vi "ILCTemperatureOnly.vi"() -> ()   [LabVIEW 2016]
uses:
  Common_RT_HealthAndStatus/RTHealthAndStatus/RTHealthAndStatus.lvclass
  MyHealthAndStatusReadFIFO/MyHealthAndStatusReadFIFO.lvclass
  D:/Code/Common_RT_FPGA/IReadU32FIFO/IReadU32FIFO.lvclass
  MyHealthAndStatusWriteFIFO/MyHealthAndStatusWriteFIFO.lvclass
  D:/Code/Common_RT_FPGA/IWriteU64FIFO/IWriteU64FIFO.lvclass
  ModbusFactory/ModbusFactory.lvclass
  D:/Code/Common_RT_Modbus/IModbusFactory/IModbusFactory.lvclass
  SubnetFactory/SubnetFactory.lvclass
  Subnet/DataTypes/SubnetSettings.ctl
  Common_RT_HPILC/DataTypes/HPSettings.ctl
  Common_RT_ILC/DataTypes/ILCSettings.ctl
  Common_RT_Modbus/IModbusFactory/IModbusFactory.lvclass
  Common_RT_MTILC/DataTypes/MTSettings.ctl
  Common_RT_MDILC/DataTypes/MDSettings.ctl
  Common_RT_MIILC/DataTypes/MISettings.ctl
  ModbusFactory/ModbusFactory.lvclass/ModbusFactory.ctl
  MyHealthAndStatusWriteFIFO/MyHealthAndStatusWriteFIFO.lvclass/MyHealthAndStatusWriteFIFO.ctl
  MyHealthAndStatusReadFIFO/MyHealthAndStatusReadFIFO.lvclass/MyHealthAndStatusReadFIFO.ctl
  Common_RT_HealthAndStatus/RTHealthAndStatus/RTHealthAndStatus.lvclass/RTHealthAndStatus.ctl
  <vilib>/Platform/TimedLoop/XDataNode/timing_clust.ctl
  <vilib>/Platform/TimedLoop/XDataNode/nitl_modes.ctl
  <vilib>/Platform/TimedLoop/XDataNode/wakeup.ctl
  Subnet/Subnet.lvclass/Subnet.ctl
  Common_RT_MTILC/MTILC/MTILC.lvclass/MTILC.ctl
  <vilib>/FPGAPlugInAG/cRIO-9038/niLvFpga_Open_cRIO-9038.vi
  <vilib>/rvi/interface/common/dynamic/niFpgaDynamicAddResources.vi
  <vilib>/FPGAPlugInAG/Dynamic/niLvFpga_Abort_Dynamic.vi
  <vilib>/FPGAPlugInAG/Dynamic/niLvFpga_Reset_Dynamic.vi
  <vilib>/FPGAPlugInAG/Dynamic/niLvFpga_Run_Dynamic.vi
  <vilib>/Utility/error.llb/Error Cluster From Error Code.vi
  <vilib>/rvi/errors/niLvFpgaAdjustHostInterfaceError.vi
  <vilib>/FPGAPlugInAG/Dynamic/niLvFpga_Close_Dynamic.vi
  <vilib>/rvi/interface/nirviOpenFPGA/nirviOpenFPGA.xnode
  FPGA Bitfiles/modbus1Port.lvbitx
  FPGA/main.vi
  <vilib>/rvi/interface/nirviMethod/nirviMethod.xnode
  <vilib>/Platform/TimedLoop/XDataNode/XDataNode.xnode
  <vilib>/rvi/interface/nirviCloseFPGA/nirviCloseFPGA.xnode
  Subnet/Subnet.lvclass
  Common_RT_ILC/RTILC.lvlib
  Common_RT_HPILC/RTHPILC.lvlib
  <vilib>/rvi/errors/niLvFpgaMergeErrorWithErrorCode.vi
  <vilib>/FPGAPlugInAG/Dynamic/niLvFpga_ReadFifo_Dynamic.vi
  Common_RT_MTILC/MTILC/MTILC.lvclass
  Common_RT_MIILC/RTMIILC.lvlib
  Common_RT_MDILC/RTMDILC.lvlib
  Common_RT_MTILC/RTMTILC.lvlib
  <vilib>/Platform/TimedLoop/XDataNode/XDNodeRunTimeDep.lvlib
panel:
  out "TimestampDelta":i64
  out "RxTimestamp":i64
  out "Avg Time Delta":dbl
  out "Min Time Delta":i64
  out "Max Time Delta":i64
  out "TxTimestamp":i64
  out "Temperature":T1(graph)
  out "InvalidCRCs":i32
  in  "Stop":bool
  out "Port 1 Status Bits":u64 format="%016b"
  out "error out":errorcluster
  out "Port 1 Frames Received":i64
  out "Port 1 Bytes Received":i64
  out "Port 1 Frames Transmitted":i64
  out "Port 1 Bytes Transmitted":i64
  # "Port 1 = Modbus"
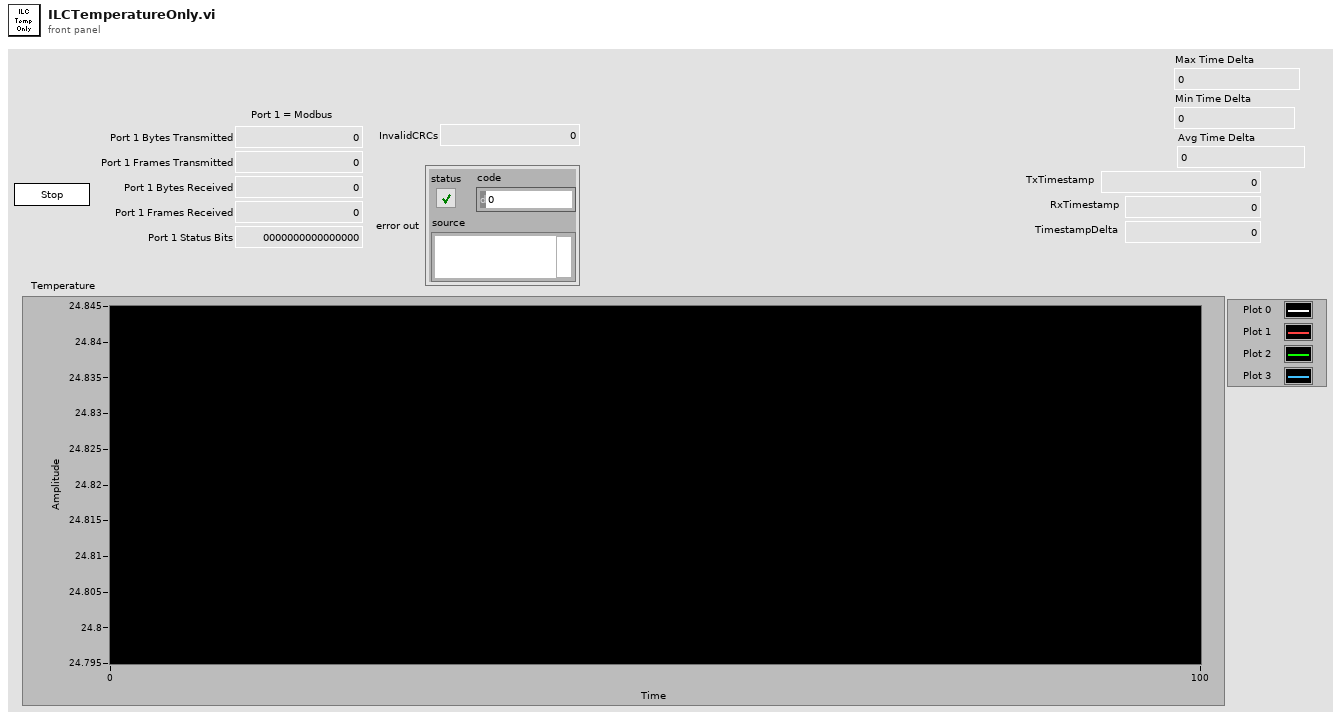
[diagram p1: front panel]
types:
  T1 = cluster{"Temperature1":sgl, "Temperature1":sgl, "Temperature1":sgl, "Temperature1":sgl}
  T2 = typedef "RTMTILC.lvlib/MTSettings.ctl" = cluster{"ILCSettings":T3, "ID":i16}
  T3 = typedef "RTILC.lvlib/ILCSettings.ctl" = cluster{"Subnet":u8, "Address":u8}
  T4 = typedef "RTHPILC.lvlib/HPSettings.ctl" = cluster{"ILCSettings":T3, "ID":i16, "ReferencePosition":i32}
  T5 = typedef "XDNodeRunTimeDep.lvlib/timing_clust.ctl" = cluster{"Expected End [f-1]":u64, "Actual End [f-1]":u64, "Finished Late? [f-1]":bool, "Expected End [i-1]":u64, "Actual End [i-1]":u64, "Finished Late? [i-1]":bool, "Expected Start [i]":u64, "Actual Start [i]":u64, "Expected Start [f]":u64, "Actual Start [f]":u64, "Source Name":string, "Structure Name":string, "Period":i64, "Deadline":i64, "Offset":i64, "Start":i64, "Priority":i32, "Timeout":i32, "Mode":T6, "Wakeup Reason":T7, "Error":errorcluster, "Source Type":string, "Secondary Source Type":string, "Global End Time":u64, "Global Start Time":u64, "Frame Duration":u64, "Iteration Duration":u64, "Assigned CPU":i32, "I/O Scan Engine Mode":u32}
  T6 = typedef "XDNodeRunTimeDep.lvlib/nitl_modes.ctl" = enum32{"No Change", "Process missed periods, maintain original phase", "Discard missed periods, maintain original phase", "Process missed periods, ignore original phase", "Discard missed periods, ignore original phase"}
  T7 = typedef "XDNodeRunTimeDep.lvlib/wakeup.ctl" = enum32{"Normal", "Aborted", "Asynchronous wakeup", "Timing source error", "Timed loop error", "Timeout"}
  T8 = typedef "SubnetSettings.ctl" = cluster{"HPs":T4[], "ModbusFactory":refnum<class "IModbusFactory.lvclass">, "Port":i32, "MTs":T2[], "MDs":T9[], "MIs":T10[]}
  T9 = typedef "RTMDILC.lvlib/MDSettings.ctl" = cluster{"ILCSettings":T3, "ID":i16}
  T10 = typedef "RTMIILC.lvlib/MISettings.ctl" = cluster{"ILCSettings":T3, "ID":i16}
  T11 = typedef "RTModbus.lvlib/RxFrame.ctl" = cluster{"Data":u8[], "Timestamp":u64}
  T12 = typedef "SubnetData.ctl" = cluster{"SubnetConstants":T13, "SubnetCommand":T16, "SubnetTelemetry":T17}
  T13 = typedef "SubnetConstants.ctl" = cluster{"Modbus":refnum<class "IModbus.lvclass">, "HPs":refnum<class "HPILC.lvclass">[], "AddressToActuator":T14[], "MTs":refnum<class "MTILC.lvclass">[], "MDs":refnum<class "MDILC.lvclass">[], "MIs":refnum<class "MIILC.lvclass">[]}
  T14 = typedef "ILCIndexData.ctl" = cluster{"ILCTypes":T15, "Index":i32}
  T15 = typedef "ILCTypes.ctl" = enum16{"Undefined", "SAA", "DAA", "HP", "MT", "MD", "MI"}
  T16 = typedef "SubnetCommand.ctl" = cluster{"BroadcastCounter":u8}
  T17 = typedef "SubnetTelemetry.ctl" = cluster{"BytesTransmitted":u32, "FramesTransmitted":u32, "BytesReceived":u32, "FramesReceived":u32, "TxInternalFIFOOverflow":bool, "InvalidInstruction":bool, "WaitForRxFrameTimeout":bool, "StartBitError":bool, "StopBitError":bool, "RxDataFIFOOverflow":bool}
  T18 = typedef "RTMTILC.lvlib/MTData.ctl" = cluster{"Constants":T19, "Telemetry":T20, "Responses":T21, "Timings":T23}
  T19 = typedef "RTMTILC.lvlib/MTConstants.ctl" = cluster{"ID":i16}
  T20 = typedef "RTMTILC.lvlib/MTTelemetry.ctl" = cluster{"Temperature":sgl[]}
  T21 = typedef "RTMTILC.lvlib/MTResponses.ctl" = cluster{"Temperature":T22}
  T22 = typedef "RTModbus.lvlib/ExceptionCodes.ctl" = u16
  T23 = typedef "RTMTILC.lvlib/MTTimings.ctl" = cluster{"Temperature":u32}
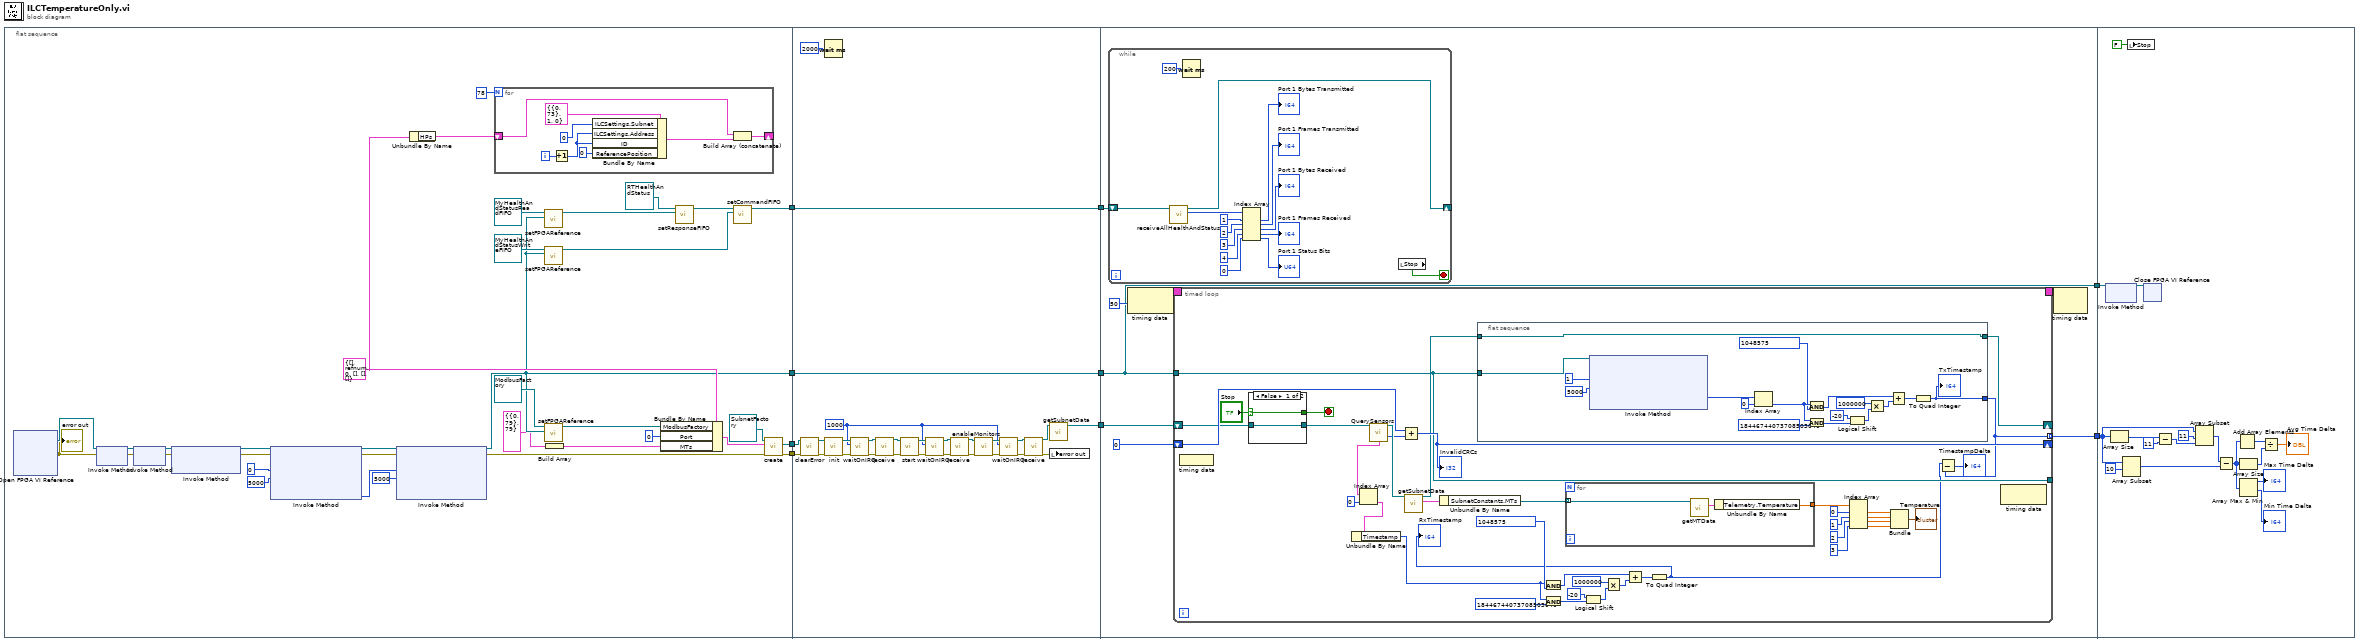
[diagram p0: block diagram]
diagram:
  n1 = flat-sequence {
    tunnel: [w19] -> w9
    tunnel: [w41] -> w6
    tunnel: [w28] -> w4
    tunnel: [w13] -> w2
    tunnel: w9 -> [w79]
    tunnel: [w79] -> w8
    tunnel: w6 -> [w77]
    tunnel: [w77] -> w5
    tunnel: w4 -> [w65]
    tunnel: [w66] -> w3
    tunnel: w2 -> [w62]
    tunnel: w8 -> [w81]
    tunnel: [w81] -> w7
    tunnel: w5 -> [w87]
    tunnel: w3 -> [w86]
    tunnel: [w80] -> w1
    tunnel: w7 -> [w187]
    tunnel: w1 -> [w185]
    frame #0 {
      w33 = T8 {"HPs"=[], "ModbusFactory"=refnum, "Port"=0, "MTs"=[], "MDs"=[], "MIs"=[]} ("SubnetSettings")
      n2 = xnode "Open FPGA VI Reference"() -> ("FPGA VI Reference Out"=w35:refnum<k20>, "error out"=w15:errorcluster)  [unwired: 2 in]
      "error out" <- w15
      n3 = xnode "Invoke Method"("FPGA VI Reference In"=w35, "error in"=w15) -> ("FPGA VI Reference Out"=w44:refnum<k20>, "error out"=w36:errorcluster)
      n4 = xnode "Invoke Method"("FPGA VI Reference In"=w44, "error in"=w36) -> ("FPGA VI Reference Out"=w21:refnum<k20>, "error out"=w18:errorcluster)
      n5 = xnode "Invoke Method"("FPGA VI Reference In"=w21, "error in"=w18) -> ("FPGA VI Reference Out"=w20:refnum<k20>, "error out"=w17:errorcluster)  [unwired: 1 in]
      n6 = xnode "Invoke Method"("FPGA VI Reference In"=w20, "error in"=w17, "Number of Elements"=u32 0, "Timeout (ms)"=5000) -> ("FPGA VI Reference Out"=w24:refnum<k20>, "error out"=w22:errorcluster, "Elements Remaining"=w25:u32)  [unwired: 1 out]
      n7 = xnode "Invoke Method"("FPGA VI Reference In"=w24, "error in"=w22, "Number of Elements"=w25, "Timeout (ms)"=5000) -> ("FPGA VI Reference Out"=w19:refnum<k20>, "error out"=w14:errorcluster)  [unwired: 2 out]
      n8 = Unbundle By Name(w33) -> ("HPs"=w16:T4[])
      n9 = for {
        N: 78 -> [_]
        shift-right: [w46] -> _
        shift-left: w16 -> [w47]
        i -> [w51]
        n10 = Increment(x=w51) -> (x+1=w45:i32)
        n11 = Bundle By Name(cluster=T4 {"ILCSettings"={"Subnet"=0, "Address"=73}, "ID"=1, "ReferencePosition"=0} ("HPSettings"), "ILCSettings.Subnet"=u8 0, "ILCSettings.Address"=w45, "ID"=w45, "ReferencePosition"=0) -> (w48:T4)
        n12 = Build Array (concatenate)(w47, w48) -> (w46:T4[])
      }
      n13 = call "setFPGAReference.vi"("FPGAReference"=w19, "MyHealthAndStatusReadFIFO in"=refnum<class "MyHealthAndStatusReadFIFO.lvclass"> refnum ("MyHealthAndStatusReadFIFO.lvclass")) -> ("MyHealthAndStatusReadFIFO out"=w39:refnum<class "MyHealthAndStatusReadFIFO.lvclass">)  [unwired: 9 in]
      n14 = call "setFPGAReference.vi"("FPGAReference"=w19, "MyHealthAndStatusWriteFIFO in"=refnum<class "MyHealthAndStatusWriteFIFO.lvclass"> refnum ("MyHealthAndStatusWriteFIFO.lvclass")) -> ("MyHealthAndStatusWriteFIFO out"=w37:refnum<class "MyHealthAndStatusWriteFIFO.lvclass">)  [unwired: 9 in]
      n15 = call "setFPGAReference.vi"("FPGAReference"=w19, "ModbusFactory in"=refnum<class "ModbusFactory.lvclass"> refnum ("ModbusFactory.lvclass")) -> ("ModbusFactory out"=w31:refnum<class "ModbusFactory.lvclass">)  [unwired: 9 in]
      n16 = Build Array(T2 {"ILCSettings"={"Subnet"=0, "Address"=79}, "ID"=79} ("MTSettings")) -> (w10:T2[])
      n17 = Bundle By Name(cluster=w33, "ModbusFactory"=w31, "Port"=0, "MTs"=w10) -> (w30:T8)
      n18 = call "setResponseFIFO.vi"("ReadU32FIFO"=w39, "RTHealthAndStatus in"=refnum<class "RTHealthAndStatus.lvclass"> refnum ("RTHealthAndStatus.lvlib:RTHealthAndStatus.lvclass")) -> ("RTHealthAndStatus out"=w42:refnum<class "RTHealthAndStatus.lvclass">)  [unwired: 9 in]
      n19 = call "setCommandFIFO.vi"("WriteU64FIFO"=w37, "RTHealthAndStatus in"=w42) -> ("RTHealthAndStatus out"=w41:refnum<class "RTHealthAndStatus.lvclass">)  [unwired: 9 in]
      n20 = call "create.vi"("error in (no error)"=w14, "SubnetSettings"=w30, "SubnetFactory in"=refnum<class "SubnetFactory.lvclass"> refnum ("SubnetFactory.lvclass")) -> ("error out"=w13:errorcluster, "Subnet"=w28:refnum<class "Subnet.lvclass">)  [unwired: 6 in, 1 out]
    }
    frame #1 {
      w53 = 1000 ("Timeout (ms)")
      n21 = call-dynamic "clearError.vi"("error in (no error)"=w62, "Subnet in"=w65) -> ("error out"=w63:errorcluster, "Subnet out"=w64:refnum<class "Subnet.lvclass">)  [unwired: 8 in]
      n22 = Wait (ms)(milliseconds to wait=u32 2000) -> ()  [unwired: 1 out]
      n23 = call-dynamic "init.vi"("error in (no error)"=w63, "Subnet in"=w64) -> ("error out"=w73:errorcluster, "Subnet out"=w76:refnum<class "Subnet.lvclass">)  [unwired: 8 in]
      n24 = call-dynamic "waitOnIRQ.vi"("error in (no error)"=w73, "Timeout (ms)"=w53, "Subnet in"=w76) -> ("error out"=w74:errorcluster, "Subnet out"=w75:refnum<class "Subnet.lvclass">)  [unwired: 7 in]
      n25 = call-dynamic "receive.vi"("Subnet in"=w75, "error in (no error)"=w74) -> ("Subnet out"=w72:refnum<class "Subnet.lvclass">, "error out"=w70:errorcluster)  [unwired: 8 in, 4 out]
      n26 = call-dynamic "start.vi"("error in (no error)"=w70, "Subnet in"=w72) -> ("error out"=w69:errorcluster, "Subnet out"=w71:refnum<class "Subnet.lvclass">)  [unwired: 8 in]
      n27 = call-dynamic "waitOnIRQ.vi"("error in (no error)"=w69, "Timeout (ms)"=w53, "Subnet in"=w71) -> ("error out"=w67:errorcluster, "Subnet out"=w68:refnum<class "Subnet.lvclass">)  [unwired: 7 in]
      n28 = call-dynamic "receive.vi"("Subnet in"=w68, "error in (no error)"=w67) -> ("Subnet out"=w61:refnum<class "Subnet.lvclass">, "error out"=w58:errorcluster)  [unwired: 8 in, 4 out]
      n29 = call-dynamic "enableMonitors.vi"("error in (no error)"=w58, "Subnet in"=w61) -> ("error out"=w57:errorcluster, "Subnet out"=w60:refnum<class "Subnet.lvclass">)  [unwired: 8 in]
      n30 = call-dynamic "waitOnIRQ.vi"("error in (no error)"=w57, "Timeout (ms)"=w53, "Subnet in"=w60) -> ("error out"=w56:errorcluster, "Subnet out"=w59:refnum<class "Subnet.lvclass">)  [unwired: 7 in]
      n31 = call-dynamic "receive.vi"("Subnet in"=w59, "error in (no error)"=w56) -> ("Subnet out"=w54:refnum<class "Subnet.lvclass">, "error out"=w55:errorcluster)  [unwired: 8 in, 4 out]
      n32 = call "getSubnetData.vi"("Subnet in"=w54) -> ("Subnet out"=w66:refnum<class "Subnet.lvclass">)  [unwired: 9 in, 1 out]
      n33 = local write "error out"(w55) -> ()
    }
    frame #2 {
      n34 = while {
        shift-right: [w169] -> _
        shift-left: w87 -> [w170]
        stop <- w157 stop-if-true
        n35 = call "receiveAllHealthAndStatus.vi"("RTHealthAndStatus in"=w170) -> ("Data"=w164:u32[], "RTHealthAndStatus out"=w169:refnum<class "RTHealthAndStatus.lvclass">)  [unwired: 8 in, 1 out]
        n36 = Wait (ms)(milliseconds to wait=u32 200) -> ()  [unwired: 1 out]
        n37 = Index Array(array=w164, index #1=1 ("index"), index #2=2 ("index"), index #3=3 ("index"), index #4=4 ("index"), index #5=0 ("index")) -> (element #1=→"Port 1 Bytes Transmitted":u32, element #2=→"Port 1 Frames Transmitted":u32, element #3=→"Port 1 Bytes Received":u32, element #4=→"Port 1 Frames Received":u32, element #5=→"Port 1 Status Bits":u32)
        n38 = local read "Stop"() -> (w157:bool)
      }
      n39 = node-c288(i64 50 ("Period")) -> (w84:T5)
      n40 = timed-loop {
        shift-right: [w106] -> _
        shift-left: w86 -> [w104]
        shift-right: [w120] -> _
        shift-left: 0 -> [w121]
        timing: w84 -> [_]
        timing-out: [_] -> w83
        tunnel: [w105] -> _
        tunnel: w81 -> [w105]
        tunnel: [w89] -> w80 mode=indexing
        stop <- w125 stop-if-true
        n41 = node-c288() -> ()  [unwired: 1 in]
        n42 = case shown="False" "Stop" {
          selector: "Stop" -> [w149 w151]
          tunnel: [w149 w151] -> w125
          tunnel: w104 -> [w150 w152]
          tunnel: [w150 w152] -> w124
          frame False {
          }
          frame True {
          }
        }
        n43 = call "QuerySensors.vi"("Subnet in"=w124) -> ("Subnet out"=w122:refnum<class "Subnet.lvclass">, "InvalidCRC"=w119:i32, "CRCIssues"=w103:T11[])  [unwired: 8 in, 4 out]
        n44 = Index Array(array=w103, index=0) -> (element=w101:T11)
        n45 = Unbundle By Name(w101) -> ("Timestamp"=w91:u64)
        n46 = Add(x=w121, y=w119) -> (x+y=w120:i32)
        "InvalidCRCs" <- w120
        n47 = call "getSubnetData.vi"("Subnet in"=w122) -> ("SubnetData"=w123:T12, "Subnet out"=w107:refnum<class "Subnet.lvclass">)  [unwired: 9 in]
        n48 = Unbundle By Name(w123) -> ("SubnetConstants.MTs"=w118:refnum<class "MTILC.lvclass">[])
        n49 = flat-sequence {
          tunnel: w107 -> [w143]
          tunnel: [w143] -> w106
          tunnel: w105 -> [w142]
          tunnel: [w137] -> w89
          frame #0 {
            n50 = xnode "Invoke Method"("FPGA VI Reference In"=w142, "Number of Elements"=u32 1, "Timeout (ms)"=5000) -> ("Data"=w139:u64[])  [unwired: 1 in, 3 out]
            n51 = Index Array(array=w139, index=0) -> (element=w136:u64)
            n52 = And(x=w136, y=u64 1048575) -> (x .and. y?=w128:u64)
            n53 = And(x=w136, y=u64 18446744073708503040) -> (x .and. y?=w133:u64)
            n54 = Logical Shift(y=i16 -20, x=w133) -> (x << y=w131:u64)
            n55 = Multiply(x=u64 1000000, y=w131) -> (x*y=w129:u64)
            n56 = Add(x=w128, y=w129) -> (x+y=w127:u64)
            n57 = To Quad Integer(1:w127) -> (0:w137:i64)
            "TxTimestamp" <- w137
          }
        }
        n58 = And(x=w91, y=u64 1048575) -> (x .and. y?=w99:u64)
        n59 = And(x=w91, y=u64 18446744073708503040) -> (x .and. y?=w94:u64)
        n60 = for {
          tunnel: w118 -> [w148] mode=indexing
          tunnel: [w146] -> w117
          n61 = call "getMTData.vi"("MTILC in"=w148) -> ("MTData"=w147:T18)  [unwired: 9 in, 1 out]
          n62 = Unbundle By Name(w147) -> ("Telemetry.Temperature"=w146:sgl[])
        }
        n63 = Logical Shift(y=i16 -20, x=w94) -> (x << y=w96:u64)
        n64 = Multiply(x=u64 1000000, y=w96) -> (x*y=w98:u64)
        n65 = Add(x=w99, y=w98) -> (x+y=w100:u64)
        n66 = To Quad Integer(1:w100) -> (0:w90:i64)
        "RxTimestamp" <- w90
        n67 = Index Array(array=w117, index #1=0 ("index"), index #2=1 ("index"), index #3=2 ("index"), index #4=3 ("index")) -> (element #1=w111:sgl, element #2=w110:sgl, element #3=w109:sgl, element #4=w108:sgl)
        n68 = Bundle("Temperature1"=w111, "Temperature1"=w110, "Temperature1"=w109, "Temperature1"=w108) -> (→"Temperature":T1)  [unwired: 1 in]
        n69 = Subtract(x=w90, y=w89) -> (x-y=→"TimestampDelta":i64)
        n70 = node-c288() -> ()  [unwired: 1 in, 1 out]
      }
      n71 = node-c288(w83) -> ()  [unwired: 1 out]
    }
    frame #3 {
      n72 = xnode "Invoke Method"("FPGA VI Reference In"=w187) -> ("FPGA VI Reference Out"=w188:refnum<k20>)  [unwired: 1 in, 1 out]
      n73 = Array Size(array=w185) -> (size(s)=w184:i32)
      n74 = Array Subset(array=w185, index=10) -> (w179:i64[])  [unwired: 1 in]
      n75 = local write "Stop"(FALSE ("Stop")) -> ()
      n76 = xnode "Close FPGA VI Reference"("FPGA VI Reference In"=w188) -> ()  [unwired: 1 in, 1 out]
      n77 = Subtract(x=w184, y=11) -> (x-y=w182:i32)
      n78 = Array Subset(array=w185, index=11, length=w182) -> (w180:i64[])
      n79 = Subtract(x=w180, y=w179) -> (x-y=w176:i64[])
      n80 = Add Array Elements(numeric array=w176) -> (sum=w175:i64)
      n81 = Array Size(array=w176) -> (size(s)=w174:i32)
      n82 = Array Max & Min(array=w176) -> (max value=→"Max Time Delta":i64, min value=→"Min Time Delta":i64)  [unwired: 2 out]
      n83 = Divide(x=w175, y=w174) -> (x/y=→"Avg Time Delta":dbl)
    }
  }
